vi "multinumericlimittest2.vi"(4 "Sequence Context":T1) -> (0 "error out":errorcluster, 1 "Test Data":T2 {"Numeric Measurement" format="%.2f"})   [LabVIEW 2010]
uses:
  Demo/LabVIEW/SupportVIs.llb/LabVIEW Test - Test Data.ctl
  <vilib>/addons/TestStand/_TSLegacy.llb/LabVIEW Test - Sequence Context.ctl
panel:
  out "Measurements":dbl[](array[numeric])=[5.0, 10.0, 15.0] format="%.2f"
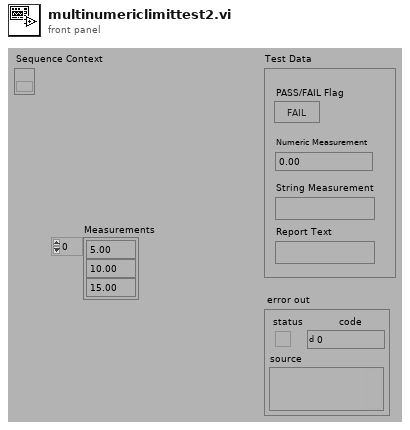
[diagram p1: front panel]
types:
  T1 = typedef "LabVIEW Test - Sequence Context.ctl" = refnum<k7>
  T2 = typedef "LabVIEW Test - Test Data.ctl" = cluster{"PASS/FAIL Flag":bool, "Numeric Measurement":dbl, "String Measurement":string, "Report Text":string}
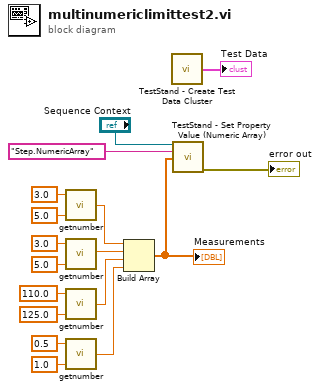
[diagram p0: block diagram]
diagram:
  n1 = call "getnumber.vi"("High Limit"=5.0, "Low Limit"=3.0) -> ("Numeric"=w13:dbl)  [unwired: 3 out]
  n2 = call "getnumber.vi"("High Limit"=5.0, "Low Limit"=3.0) -> ("Numeric"=w10:dbl)  [unwired: 3 out]
  n3 = call "getnumber.vi"("High Limit"=125.0, "Low Limit"=110.0) -> ("Numeric"=w7:dbl)  [unwired: 3 out]
  n4 = call "getnumber.vi"("High Limit"=1.0, "Low Limit"=0.5) -> ("Numeric"=w2:dbl)  [unwired: 3 out]
  n5 = Build Array(w13, w10, w7, w2) -> (w1:dbl[])
  "Measurements" <- w1
  n6 = call "TestStand - Create Test Data Cluster.vi"() -> ("Test Data"=→"Test Data":T2)  [unwired: 4 in]
  n7 = call <vilib>:"TestStand - Set Property Value (Numeric Array).vi"("Sequence Context In"="Sequence Context", "Lookup String"="Step.NumericArray", "New Value"=w1) -> ("error out"=→"error out":errorcluster)  [unwired: 2 in, 10 out]
